vi "JHOC Top Stack.vi"(2 "State Stack (in)":T1[](array[typedef])) -> (0 "State Stack (out)":T1[](array[typedef]), 1 "State 4":T1=enum."Calculate 6 Field/Int Rot Matrix")   [LabVIEW 2013]
uses:
  JHOC state.ctl
panel:
  # "Top Stack\nVER 1.0 AAM 10th April 2002\n\nThis VI removes the top element of the state stack \nand returns the remaining elements in the stack"
  # "Copyright Americo A. Migliaccio (c) 2002 All Rights Reserved by Author"
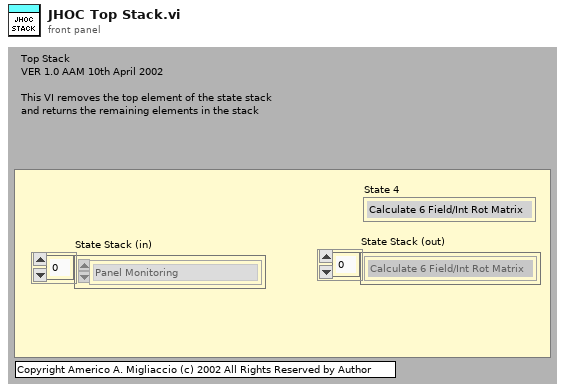
[diagram p1: front panel]
types:
  T1 = typedef "JHOC state.ctl" = enum16{"Panel Monitoring", "Calculate 6 Field/Int Rot Matrix", "SubSample", "Initialize", "Read 6 Field/Int Calibration File", "Read 6 Field/Int Data File", "Sort 6 Field/Int Channels", "Export Channels", "Stop", "Quit"}
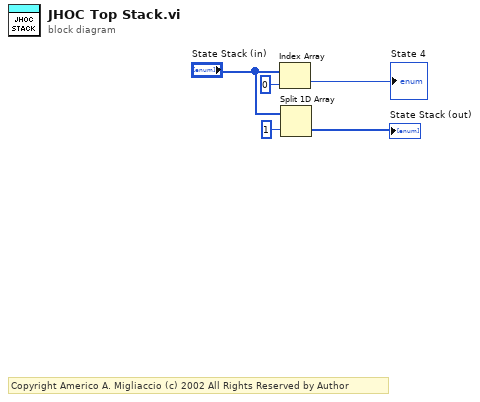
[diagram p0: block diagram]
diagram:
  # "Copyright Americo A. Migliaccio (c) 2002 All Rights Reserved by Author"
  n1 = Index Array(array="State Stack (in)", index=0) -> (element=→"State 4":T1)
  n2 = Split 1D Array(array="State Stack (in)", index=1) -> (second subarray=→"State Stack (out)":T1[])  [unwired: 1 out]
